vi "SN Sort.vi"(7 "Array In":string[](array[string])) -> (8 "Array Out":string[](array[string]))   [LabVIEW 2019]
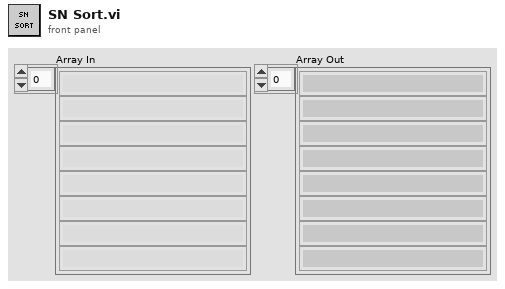
[diagram p1: front panel]
types:
  T1 = cluster{string, string, string, string, string}[]
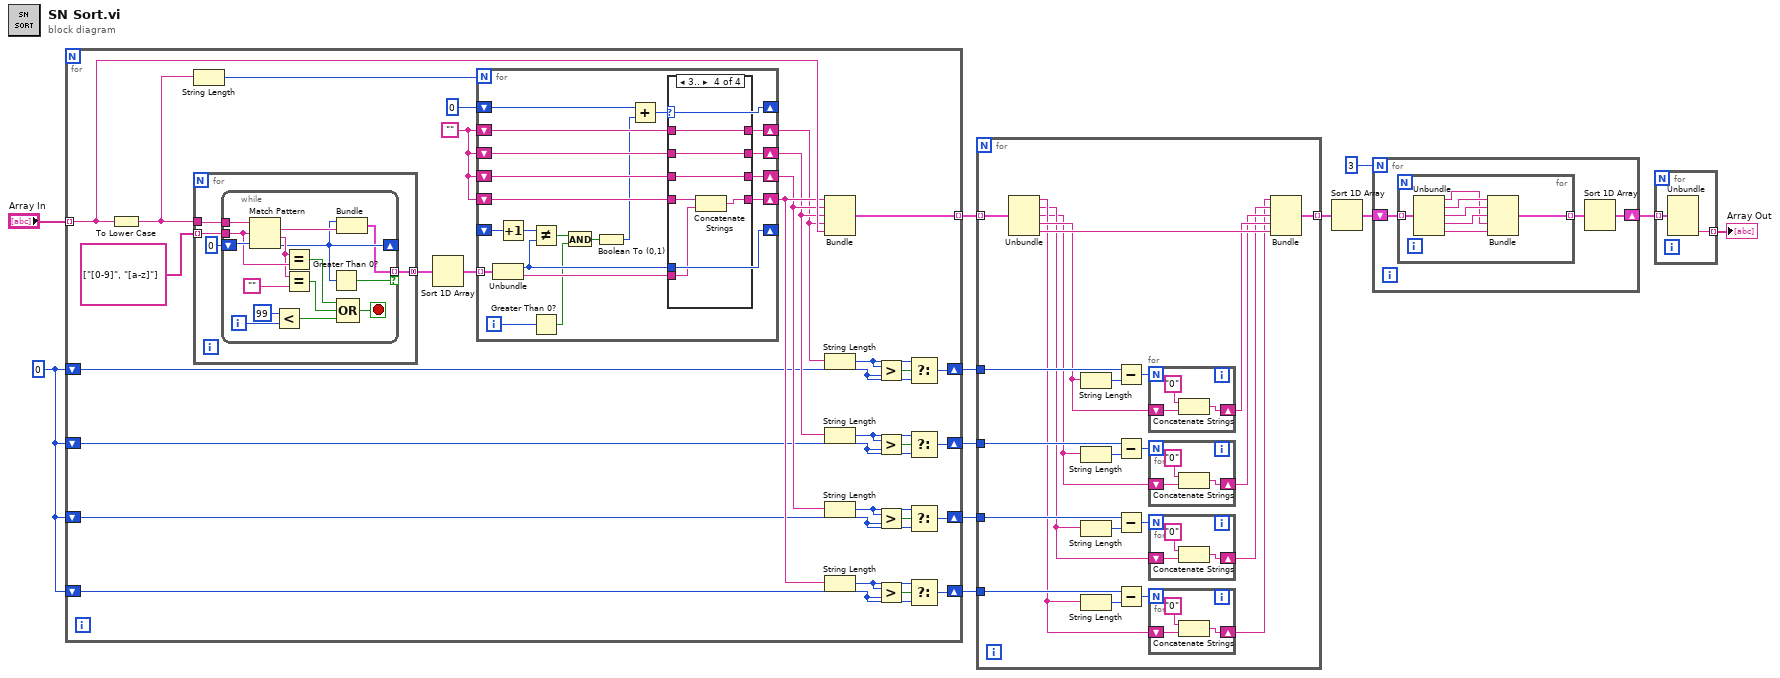
[diagram p0: block diagram]
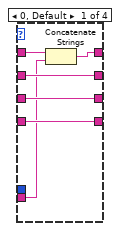
[diagram p2: hidden frame]
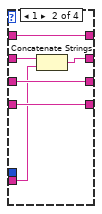
[diagram p3: hidden frame]
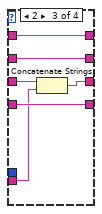
[diagram p4: hidden frame]
diagram:
  w10 = 0
  n1 = for {
    tunnel: [w34] -> w12 mode=indexing
    tunnel: "Array In" -> [w33] mode=indexing
    shift-right: [w18] -> w8
    shift-left: w10 -> [w19]
    shift-right: [w16] -> w7
    shift-left: w10 -> [w21]
    shift-right: [w17] -> w6
    shift-left: w10 -> [w20]
    shift-right: [w25] -> w9
    shift-left: w10 -> [w26]
    w35 = ""
    n2 = To Lower Case(string=w33) -> (all lower case string=w40:string)
    n3 = String Length(string=w40) -> (length=w37:i32)
    n4 = for {
      tunnel: string[] ["[0-9]", "[a-z]"] -> [w88] mode=indexing
      tunnel: w40 -> [w89]
      tunnel: [w86] -> w39 mode=concatenating
      n5 = while {
        tunnel: w89 -> [w104]
        tunnel: w88 -> [w99]
        shift-right: [w91] -> _
        shift-left: 0 ("offset past match") -> [w103]
        tunnel: [w90] -> w86 mode=indexing if=w93
        i -> [w101]
        stop <- w94 stop-if-true
        n6 = Match Pattern(string=w104, regular expression=w99, offset (0)=w103) -> (match substring=w92:string, after substring=w98:string, offset past match=w91:i32)  [unwired: 1 out]
        n7 = Less?(x=99, y=w101) -> (x < y?=w100:bool)
        n8 = Equal?(x=w98, y=w99) -> (x = y?=w95:bool)
        n9 = Equal?(x=w98, y="") -> (x = y?=w96:bool)
        n10 = Greater Than 0?(x=w91) -> (x > 0?=w93:bool)
        n11 = Bundle("offset past match"=w91, w92) -> (w90:cluster{"offset past match":i32, string})  [unwired: 1 in]
        n12 = Compound Arithmetic op=OR(w95, w96, w100) -> (w94:bool)
      }
    }
    n13 = Sort 1D Array(array=w39) -> (sorted array=w38:cluster{"offset past match":i32, string}[])
    n14 = for {
      N: w37 -> [_]
      tunnel: w38 -> [w61] mode=indexing
      shift-right: [w47] -> _
      shift-left: 0 -> [w48]
      shift-right: [w53] -> w29
      shift-left: w35 -> [w60]
      shift-right: [w56] -> w30
      shift-left: w35 -> [w59]
      shift-right: [w55] -> w31
      shift-left: w35 -> [w58]
      shift-right: [w54] -> w32
      shift-left: w35 -> [w57]
      shift-right: [w50] -> _
      shift-left: _ -> [w52]
      i -> [w43]
      n15 = Unbundle(w61) -> ("offset past match"=w50:i32, w46:string)
      n16 = Increment(x=w52) -> (x+1=w51:i32)
      n17 = Not Equal?(x=w51, y=w50) -> (x != y?=w45:bool)
      n18 = Greater Than 0?(x=w43) -> (x > 0?=w44:bool)
      n19 = And(x=w45, y=w44) -> (x .and. y?=w42:bool)
      n20 = Boolean To (0,1)(Boolean=w42) -> (0, 1=w49:i16)
      n21 = Add(x=w48, y=w49) -> (x+y=w47:i32)
      n22 = case shown="3.." w47 {
        tunnel: w50 -> [_ _ _ _]
        tunnel: w60 -> [w64 w69 w78 w85]
        tunnel: w59 -> [w67 w71 w75 w84]
        tunnel: w58 -> [w66 w73 w77 w82]
        tunnel: w57 -> [w65 w72 w79 w83]
        tunnel: [w67 w70 w75 w84] -> w56
        tunnel: [w66 w73 w76 w82] -> w55
        tunnel: [w65 w72 w79 w81] -> w54
        tunnel: [w63 w69 w78 w85] -> w53
        tunnel: w46 -> [w62 w68 w74 w80]
        frame 0, Default {
          n23 = Concatenate Strings(w64, w62) -> (w63:string)
        }
        frame 1 {
          n24 = Concatenate Strings(w71, w68) -> (w70:string)
        }
        frame 2 {
          n25 = Concatenate Strings(w77, w74) -> (w76:string)
        }
        frame 3.. {
          n26 = Concatenate Strings(w83, w80) -> (w81:string)
        }
      }
    }
    n27 = Bundle(w32, w31, w30, w29, w33) -> (w34:cluster{string, string, string, string, string})  [unwired: 1 in]
    n28 = String Length(string=w29) -> (length=w28:i32)
    n29 = String Length(string=w30) -> (length=w15:i32)
    n30 = String Length(string=w31) -> (length=w14:i32)
    n31 = String Length(string=w32) -> (length=w13:i32)
    n32 = Greater?(x=w28, y=w26) -> (0:w27:bool)
    n33 = Greater?(x=w15, y=w19) -> (0:w22:bool)
    n34 = Greater?(x=w14, y=w21) -> (0:w24:bool)
    n35 = Greater?(x=w13, y=w20) -> (0:w23:bool)
    n36 = Select(t=w28, s=w27, f=w26) -> (s? t:f=w25:i32)
    n37 = Select(t=w15, s=w22, f=w19) -> (s? t:f=w18:i32)
    n38 = Select(t=w14, s=w24, f=w21) -> (s? t:f=w16:i32)
    n39 = Select(t=w13, s=w23, f=w20) -> (s? t:f=w17:i32)
  }
  n40 = for {
    tunnel: w12 -> [w127] mode=indexing
    tunnel: w8 -> [w119]
    tunnel: w9 -> [w125]
    tunnel: w7 -> [w114]
    tunnel: w6 -> [w113]
    tunnel: [w105] -> w1 mode=indexing
    n41 = Unbundle(w127) -> (w108:string, w107:string, w106:string, w122:string, w126:string)
    n42 = String Length(string=w122) -> (length=w124:i32)
    n43 = String Length(string=w106) -> (length=w120:i32)
    n44 = String Length(string=w107) -> (length=w115:i32)
    n45 = String Length(string=w108) -> (length=w118:i32)
    n46 = Subtract(x=w125, y=w124) -> (x-y=w123:i32)
    n47 = Subtract(x=w119, y=w120) -> (x-y=w121:i32)
    n48 = Subtract(x=w114, y=w115) -> (x-y=w116:i32)
    n49 = Subtract(x=w113, y=w118) -> (x-y=w117:i32)
    n50 = for {
      N: w123 -> [_]
      shift-right: [w138] -> w112
      shift-left: w122 -> [w139]
      n51 = Concatenate Strings("0", w139) -> (w138:string)
    }
    n52 = for {
      N: w121 -> [_]
      shift-right: [w135] -> w111
      shift-left: w106 -> [w136]
      n53 = Concatenate Strings("0", w136) -> (w135:string)
    }
    n54 = for {
      N: w116 -> [_]
      shift-right: [w132] -> w110
      shift-left: w107 -> [w133]
      n55 = Concatenate Strings("0", w133) -> (w132:string)
    }
    n56 = for {
      N: w117 -> [_]
      shift-right: [w129] -> w109
      shift-left: w108 -> [w130]
      n57 = Concatenate Strings("0", w130) -> (w129:string)
    }
    n58 = Bundle(w109, w110, w111, w112, w126) -> (w105:cluster{string, string, string, string, string})  [unwired: 1 in]
  }
  n59 = Sort 1D Array(array=w1) -> (sorted array=w4:T1)
  n60 = for {
    N: 3 -> [_]
    shift-right: [w140] -> w3
    shift-left: w4 -> [w142]
    n61 = for {
      tunnel: w142 -> [w149] mode=indexing
      tunnel: [w147] -> w141 mode=indexing
      n62 = Unbundle(w149) -> (w143:string, w144:string, w145:string, w146:string, w148:string)
      n63 = Bundle(w144, w145, w146, w143, w148) -> (w147:cluster{string, string, string, string, string})  [unwired: 1 in]
    }
    n64 = Sort 1D Array(array=w141) -> (sorted array=w140:T1)
  }
  n65 = for {
    tunnel: w3 -> [w151] mode=indexing
    tunnel: [w150] -> w2 mode=indexing
    n66 = Unbundle(w151) -> (w150:string)  [unwired: 4 out]
  }
  "Array Out" <- w2
